vi "Dataset.vi"(8 "error in (no error)":errorcluster, 9 "Dataset Trans Id":T1, 10 "Data In":dbl[](array[numeric]), 11 "DAO Actions":T5) -> (0 "error out":errorcluster, 2 "Data Out":dbl[](array[numeric]))   [LabVIEW 2009]
uses:
  Data Access Objects/Metadata/DAO Actions.ctl
  Transactions/Dataset Transaction Id.ctl
  Transactions/Dataset Source.ctl
  Transactions/Dataset Type.ctl
  Apps/Yes No Button.ctl
panel:
  out "not found":bool
  out "Label":string
  out "Dataset":variant
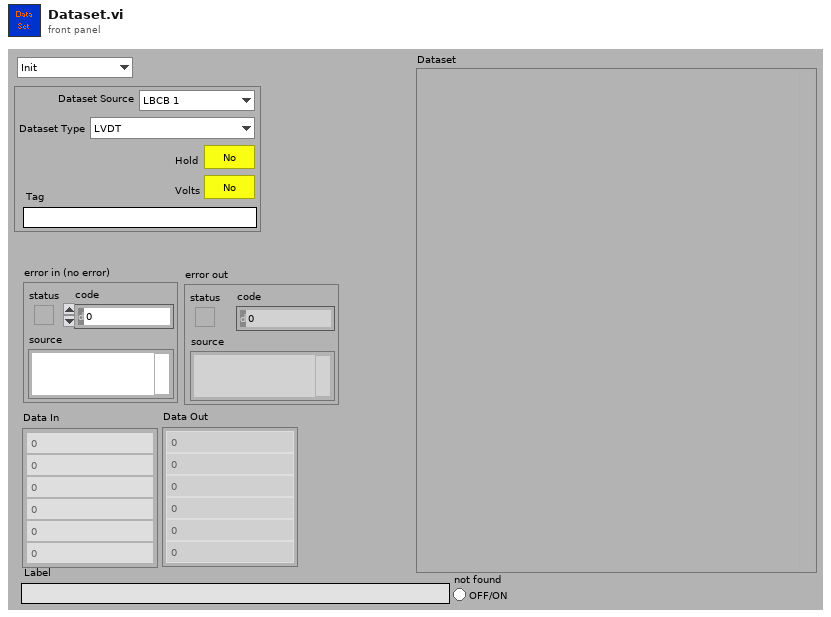
[diagram p1: front panel]
types:
  T1 = typedef "Dataset Transaction Id.ctl" = cluster{"Dataset Source":T2, "Dataset Type":T3, "Hold":T4, "Volts":T4, "Tag":string}
  T2 = typedef "Dataset Source.ctl" = enum16{"LBCB 1", "LBCB 2", "Combined", "External Sensors"}
  T3 = typedef "Dataset Type.ctl" = enum16{"LVDT", "Load Cell", "Actuator Command", "Servo Error", "Displacement Command", "Displacement", "Force"}
  T4 = typedef "Yes No Button.ctl" = bool
  T5 = typedef "DAO Actions.ctl" = enum16{"Init", "Get", "Set"}
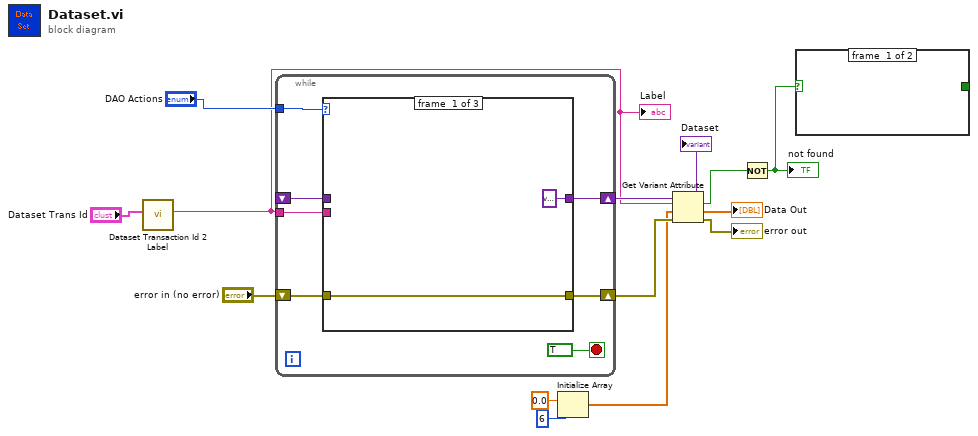
[diagram p0: block diagram]
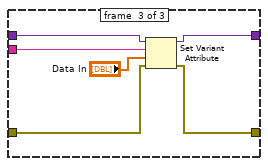
[diagram p4: hidden frame]
diagram:
  n1 = call "Dataset Transaction Id 2 Label.vi"("Dataset Trans Id"="Dataset Trans Id") -> ("Label"=w4:string)  [unwired: 10 in]
  "Label" <- w4
  n2 = while {
    tunnel: "DAO Actions" -> [w19]
    tunnel: w4 -> [w18]
    shift-right: [w16] -> w8
    shift-left: _ -> [w17]
    shift-right: [w14] -> w7
    shift-left: "error in (no error)" -> [w15]
    stop <- TRUE stop-if-true
    n3 = case shown="\"Get\"" w19 {
      tunnel: w18 -> [_ _ w29]
      tunnel: w17 -> [_ w24 w28]
      tunnel: [variant w24 w27] -> w16
      tunnel: w15 -> [w22 w23 w26]
      tunnel: [w22 w23 w25] -> w14
      frame #0 {
      }
      frame #1 {
      }
      frame #2 {
        n4 = Set Variant Attribute(Variant=w28, name=w29, value="Data In", error in=w26) -> (Variant out=w27:variant, error out=w25:errorcluster)  [unwired: 1 out]
      }
    }
  }
  "Dataset" <- w8
  n5 = Initialize Array(0.0 ("element"), 6 ("dimension size")) -> (w5:dbl[])
  n6 = Get Variant Attribute(Variant=w8, name=w4, default value (empty Variant)=w5, error in=w7) -> (found=w2:bool, value=→"Data Out":dbl[], error out=→"error out":errorcluster)  [unwired: 1 out]
  n7 = Not(x=w2) -> (.not. x?=w1:bool)
  "not found" <- w1
  n8 = case shown="True" w1 {
    selector: w1 -> [_ w31]
    tunnel: [_ w31] -> _
    frame #0 {
    }
    frame #1 {
    }
  }
